vi "Test2_2.vi"(0 "Instrument VISA in":T1={"AWG VISA"="AGTMY51400121", "Oscilloscope  VISA "="labosc4", "Integration Board IP"="172.16.7.43", "connection ID"=refnum, "report out"=refnum, "report file path"=path "C:/CTA/LevelTriggerBoardTest/TestsData/sumtrigger_delay"}, 5 "L1 min values":i32[](array[numeric]), 7 "channel array":i32[](array[numeric])=[0, 1, 2, 3, 5, 6, 7], 11 "error in":errorcluster, 13 "Cycles Burst":i32=10000) -> (4 "Instrument VISA out":T1, 6 "ATT values":dbl[][](array[numeric]), 8 "XY Graph":cluster{"Y":dbl[], "Y":dbl[]}[](graph), 15 "error out":errorcluster)   [LabVIEW 2009]
uses:
  <vilib>/Utility/NIReport.llb/NI_report.lvclass
  <instrlib>/Agilent 81150/Agilent 81150.lvlib
  <vilib>/Analysis/NI_AALPro.lvlib
panel:
  out "IPR_Address":i32
  out "L1 Address":i32=17
  in  "L1 version":bool
  in  "Report Enable":bool=TRUE
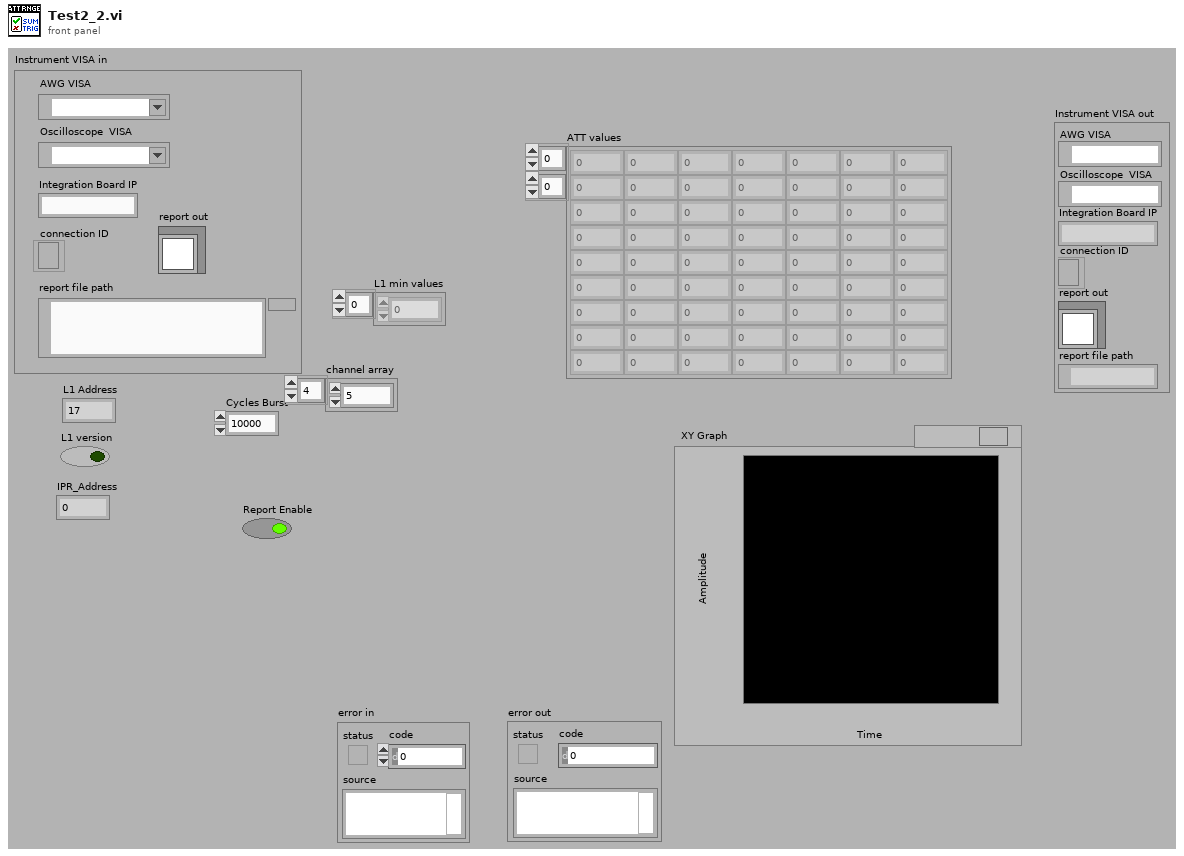
[diagram p1: front panel]
types:
  T1 = cluster{"AWG VISA":refnum<visa-resource-name>, "Oscilloscope  VISA ":refnum<visa-resource-name>, "Integration Board IP":string, "connection ID":refnum<k5>, "report out":refnum<class "NI_report.lvclass">, "report file path":path}
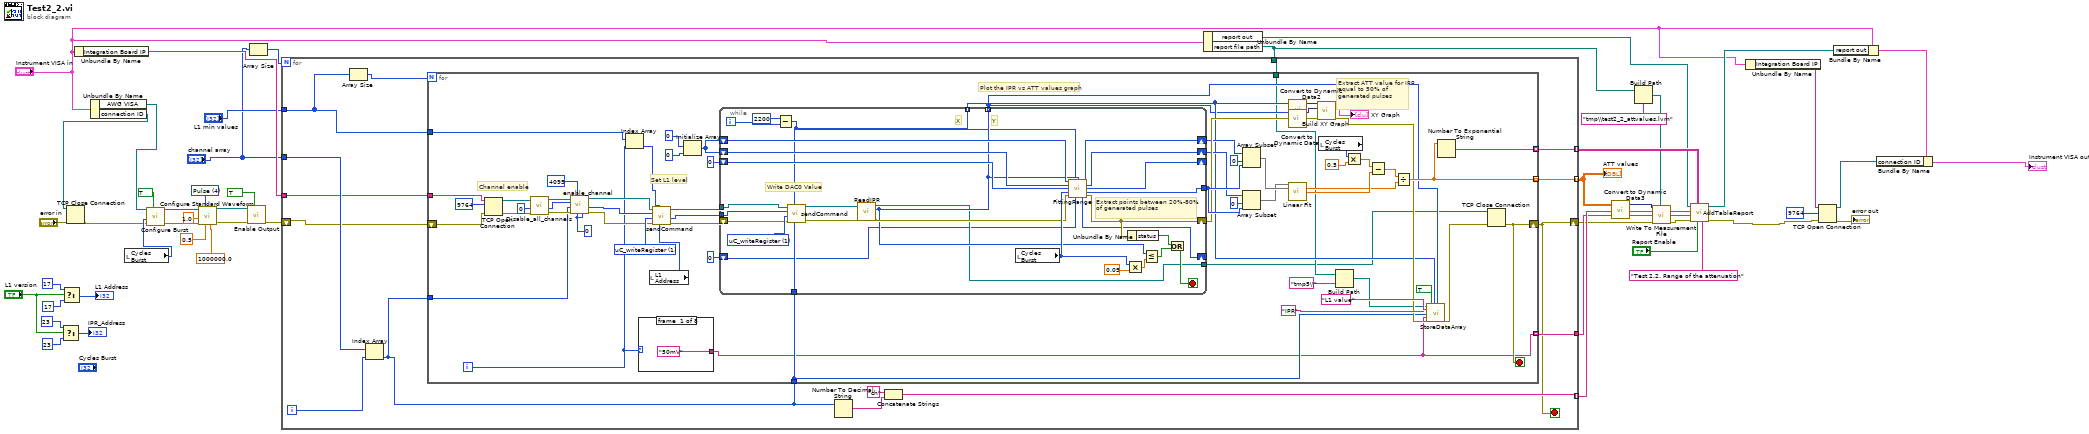
[diagram p0: block diagram]
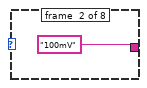
[diagram p2: hidden frame]
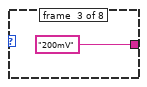
[diagram p3: hidden frame]
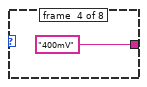
[diagram p4: hidden frame]
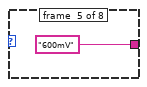
[diagram p5: hidden frame]
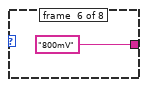
[diagram p6: hidden frame]
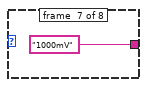
[diagram p7: hidden frame]
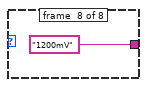
[diagram p8: hidden frame]
diagram:
  w48 = u16 4 items=["Sine", "Square", "Ramp Up", "Ramp Down", "Pulse", "Noise", "DC"] ("Waveform (0: Sine)")
  n1 = Select(t=23 ("Address"), s="L1 version", f=23 ("Address")) -> (s? t:f=→"IPR_Address":i32)
  n2 = Select(t=17 ("Address"), s="L1 version", f=17 ("Address")) -> (s? t:f=→"L1 Address":i32)
  n3 = Unbundle By Name("Instrument VISA in") -> ("Integration Board IP"=w23:string)
  n4 = Unbundle By Name("Instrument VISA in") -> ("AWG VISA"=w39:refnum<visa-resource-name>, "connection ID"=w19:refnum<k5>)
  n5 = TCP Close Connection(connection ID=w19, error in (no error)="error in") -> (error out=w21:errorcluster)  [unwired: 1 in, 1 out]
  n6 = local read "Cycles Burst"() -> (w40:i32)
  n7 = call <instrlib>:"Configure Burst.vi"("Enable Burst (F: Disable)"=TRUE, "error in (no error)"=w21, "Burst Count (2)"=w40, "VISA resource name"=w39) -> ("error out"=w45:errorcluster, "VISA resource name out"=w46:refnum<visa-resource-name>)  [unwired: 6 in]
  n8 = call <instrlib>:"Configure Standard Waveform.vi"("Frequency (1000.0 Hz)"=1000000.0, "DC Offset (0.0 Volts)"=0.5, "Waveform (0: Sine)"=w48, "error in (no error)"=w45, "Amplitude (1.0 Vpp)"=1.0, "VISA resource name"=w46) -> ("error out"=w44:errorcluster, "VISA resource name out"=w43:refnum<visa-resource-name>)  [unwired: 4 in]
  n9 = call <instrlib>:"Enable Output.vi"("Enable Output (T: Enable)"=TRUE, "error in (no error)"=w44, "VISA resource name"=w43) -> ("error out"=w38:errorcluster)  [unwired: 7 in, 1 out]
  n10 = Array Size(array="channel array") -> (size(s)=w11:i32)
  n11 = Unbundle By Name("Instrument VISA in") -> ("report out"=w34:refnum<class "NI_report.lvclass">, "report file path"=w3:path)
  n12 = for {
    N: w11 -> [_]
    tunnel: [w64] -> w2 mode=indexing
    shift-right: [w53] -> w6
    shift-left: w38 -> [w51]
    tunnel: [w63] -> w37 mode=indexing
    tunnel: [w60] -> w32 mode=indexing
    tunnel: [w59] -> w31
    tunnel: "L1 min values" -> [w55]
    tunnel: w23 -> [w50]
    tunnel: "channel array" -> [w57]
    tunnel: w3 -> [w56]
    i -> [w58]
    stop <- w53 stop-if-true
    n13 = Array Size(array=w55) -> (size(s)=w54:i32)
    n14 = Index Array(array=w57, index=w58) -> (element=w52:i32)
    n15 = for {
      N: w54 -> [_]
      tunnel: w52 -> [w96]
      tunnel: [w103] -> w64 mode=indexing
      shift-right: [w85] -> w53
      shift-left: w51 -> [w71]
      tunnel: w55 -> [w104]
      tunnel: [w102] -> w63 mode=indexing
      tunnel: [w66] -> w59 mode=indexing
      tunnel: w56 -> [w87]
      tunnel: w52 -> [w72]
      tunnel: w50 -> [w69]
      i -> [w65]
      stop <- w85 stop-if-true
      w81 = 0 ("V clip")
      w107 = u16 1 items=["sendCommand"=9, "FPGA_writeRegister"=3, "FPGA_readRegister"=2, "uC_writeRegister"=1, "uC_readRegister"=0] ("Action")
      # "Channel enable"
      # "Set L1 level"
      # "Extract ATT value for IPR equal to 50% of generated pulses"
      # "Plot the IPR vs ATT values graph"
      n16 = TCP Open Connection(address=w69, remote port or service name=u16 9764, error in (no error)=w71) -> (connection ID=w78:refnum<k5>, error out=w77:errorcluster)  [unwired: 2 in]
      n17 = call "Disable_all_channels.vi"("error in"=w77, "id_in"=0, "connection ID"=w78) -> ("error out"=w76:errorcluster, "id_out"=w80:i32, "connection ID out"=w79:refnum<k5>)  [unwired: 6 in]
      n18 = call "enable_channel.vi"("Delay"=w81, "V clip"=w81, "V att"=4095, "error in"=w76, "Channel"=w72, "id_in"=w80, "connection ID"=w79) -> ("error out"=w70:errorcluster, "id_out"=w73:i32, "connection ID out"=w74:refnum<k5>)  [unwired: 2 in]
      n19 = Index Array(array=w104, index=w65) -> (element=w67:i32)
      n20 = case shown="7" w65 {
        tunnel: ["50mV" ("regular expression") "100mV" ("regular expression") "200mV" ("regular expression") "400mV" ("regular expression") "600mV" ("regular expression") "800mV" ("regular expression") "1000mV" ("regular expression") "1200mV" ("regular expression")] -> w66
        frame #0 {
        }
        frame #1 {
        }
        frame #2 {
        }
        frame #3 {
        }
        frame #4 {
        }
        frame #5 {
        }
        frame #6 {
        }
        frame #7 {
        }
      }
      n21 = local read "L1 Address"() -> (w108:i32)
      n22 = call "sendCommand.vi"("Address"=w108, "Data"=w67, "error in"=w70, "Action"=w107, "id_in"=w73, "connection ID"=w74) -> ("error out"=w105:errorcluster, "id_out"=w90:i32, "connection ID out"=w106:refnum<k5>)  [unwired: 1 in, 2 out]
      n23 = Initialize Array(0 ("element"), 0 ("dimension size")) -> (w120:i32[])
      n24 = while {
        tunnel: w96 -> [w161]
        tunnel: [w141] -> w91 mode=indexing
        tunnel: [w138] -> w92 mode=indexing
        shift-right: [w157] -> w95
        shift-left: w120 -> [w155]
        shift-right: [w156] -> w94
        shift-left: w120 -> [w154]
        shift-right: [w147] -> w109
        shift-left: w105 -> [w160]
        shift-right: [w152] -> _
        shift-left: 0 ("Array Pointer out") -> [w153]
        tunnel: [w151] -> w116
        tunnel: w106 -> [w149]
        tunnel: [w137] -> w84
        tunnel: w90 -> [w136]
        shift-right: [w134] -> _
        shift-left: 0 ("State machine") -> [w135]
        i -> [w140]
        stop <- w145 stop-if-true
        w162 = u16 1 items=["sendCommand"=9, "FPGA_writeRegister"=3, "FPGA_readRegister"=2, "uC_writeRegister"=1, "uC_readRegister"=0] ("Action")
        # "Extract points between 20%-80% of generated pulses"
        # "Write DAC0 Value"
        # "Y"
        # "X"
        n25 = Subtract(x=2200, y=w140) -> (x-y=w138:i32)
        n26 = call "sendCommand.vi"("Address"=w161, "Data"=w138, "error in"=w160, "Action"=w162, "id_in"=w136, "connection ID"=w149) -> ("error out"=w144:errorcluster, "connection ID out"=w143:refnum<k5>)  [unwired: 1 in, 3 out]
        n27 = call "ReadIPR.vi"("error in"=w144, "connection ID"=w143) -> ("error out"=w142:errorcluster, "IPR value"=w141:i32, "connection ID out"=w137:refnum<k5>)  [unwired: 7 in]
        n28 = local read "Cycles Burst"() -> (w150:i32)
        n29 = call "FittingRange.vi"("Array in (X)"=w155, "L0 DAC"=w138, "IPR"=w141, "Array in (Y)"=w154, "Array Pointer in"=w153, "Cycles Burst"=w150, "error in"=w142, "State machine"=w135) -> ("Array out (X)"=w157:i32[], "Array out (Y)"=w156:i32[], "Array Pointer out"=w152:i32, "N_Array Elements"=w151:i32, "State machine"=w134:i32, "error out"=w147:errorcluster)  [unwired: 2 in]
        n30 = Multiply(x=w150, y=0.05) -> (x*y=w158:dbl)
        n31 = Unbundle By Name(w147) -> ("status"=w146:bool)
        n32 = Less Or Equal?(x=w141, y=w158) -> (x <= y?=w148:bool)
        n33 = Or(x=w146, y=w148) -> (x .or. y?=w145:bool)
      }
      n34 = Array Subset(array=w94, index=0, length=w116) -> (w93:i32[])
      n35 = Array Subset(array=w95, index=0, length=w116) -> (w98:i32[])
      n36 = call "Convert to Dynamic Data"("Array"=w91) -> ("Dynamic Data Type"=w124:dynamicdata)  [unwired: 3 in]
      n37 = call <vilib>:"Linear Fit.vi"("Y"=w93, "X"=w98) -> ("slope"=w110:dbl, "intercept"=w112:dbl)  [unwired: 9 in, 3 out]
      n38 = call "Convert to Dynamic Data2"("Array"=w92) -> ("Dynamic Data Type"=w123:dynamicdata)  [unwired: 3 in]
      n39 = call "Build XY Graph"("error in (no error)"=w109, "Y Input"=w124, "X Input"=w123) -> ("error out"=w97:errorcluster, "XY Graph"=→"XY Graph":cluster{"Y":dbl[], "Y":dbl[]}[])  [unwired: 7 in]
      n40 = local read "Cycles Burst"() -> (w115:i32)
      n41 = Build Path(base path=w87, name or relative path="tmp5\\") -> (appended path=w89:path)
      n42 = Multiply(x=w115, y=0.5) -> (x*y=w113:dbl)
      n43 = Subtract(x=w113, y=w112) -> (x-y=w111:dbl)
      n44 = Divide(x=w111, y=w110) -> (x/y=w103:dbl)
      n45 = call "StoreDataArray.vi"("Base path"=w89, "X Signal Name"="L1 value", "Y Signal Name"="IPR", "Channel number"=w96, "Si"=w66, "error in"=w97, "Save test data"=TRUE, "X Array"=w92, "Y Array"=w91) -> ("error out"=w86:errorcluster)  [unwired: 10 in]
      n46 = Number To Exponential String(number=w103) -> (E-format string=w102:string)  [unwired: 3 in]
      n47 = TCP Close Connection(connection ID=w84, error in (no error)=w86) -> (error out=w85:errorcluster)  [unwired: 1 in, 1 out]
    }
    n48 = Number To Decimal String(number=w52) -> (decimal integer string=w61:string)  [unwired: 1 in]
    n49 = Concatenate Strings("ch" ("string"), w61) -> (w60:string)
  }
  "ATT values" <- w2
  n50 = call "Convert to Dynamic Data3"("2D Array"=w2) -> ("Dynamic Data Type"=w4:dynamicdata)  [unwired: 3 in]
  n51 = Build Path(base path=w3, name or relative path="tmp\\test2_2_attvalues.lvm") -> (appended path=w7:path)
  n52 = call "Write To Measurement File"("Signals"=w4, "error in (no error)"=w6, "Filename"=w7) -> ("error out"=w5:errorcluster)  [unwired: 14 in, 2 out]
  n53 = call "AddTableReport.vi"("Table title"="Test 2.2. Range of the attenuation", "Report Enable"="Report Enable", "Data"=w37, "error in"=w5, "Columns"=w31, "Rows"=w32, "report in"=w34) -> ("error out"=w1:errorcluster, "report out"=w33:refnum<class "NI_report.lvclass">)  [unwired: 3 in]
  n54 = Unbundle By Name("Instrument VISA in") -> ("Integration Board IP"=w17:string)
  n55 = TCP Open Connection(address=w17, remote port or service name=u16 9764, error in (no error)=w1) -> (connection ID=w16:refnum<k5>, error out=→"error out":errorcluster)  [unwired: 2 in]
  n56 = Bundle By Name(cluster="Instrument VISA in", "report out"=w33) -> (w14:T1)
  n57 = Bundle By Name(cluster=w14, "connection ID"=w16) -> (→"Instrument VISA out":T1)
